vi "NodeID to Section Pointer.vi"(8 "error in (no error)":errorcluster, 11 "nodeID in":T1 format="%.0x") -> (0 "error out":errorcluster, 2 "BaseNodeType out":refnum<k24>, 3 "nodeID out":T1 format="%.0x")   [LabVIEW 2023, in "Instrument Addon Scripting API.lvlib"]
uses:
  Instrument Addon Scripting API.lvlib
  <vilib>/NI VeriStand/Custom Device API/Custom Device Item Ref.ctl
  NationalInstruments.VeriStand.SystemStorage
  NationalInstruments.VeriStand.SystemDefinitionAPI
  <vilib>/NI VeriStand/Custom Device API/Custom Device API.lvlib
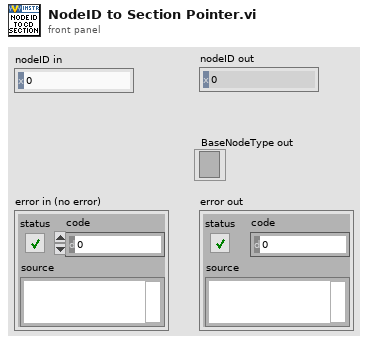
[diagram p1: front panel]
types:
  T1 = typedef "Custom Device API.lvlib/Custom Device Item Ref.ctl" = u64
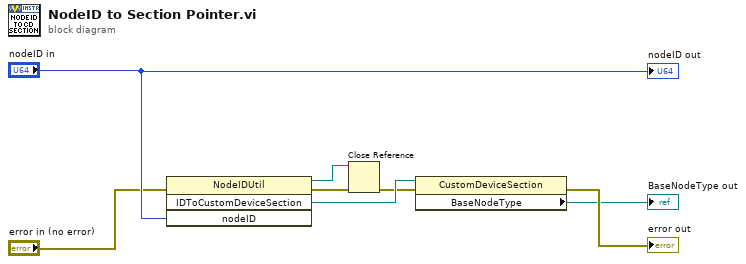
[diagram p0: block diagram]
diagram:
  n1 = invoke class="NodeIDUtil" method="IDToCustomDeviceSection"(error in="error in (no error)", "nodeID"="nodeID in") -> (reference out=w2:refnum<k24>, error out=w3:errorcluster, "IDToCustomDeviceSection"=w4:refnum<k24>)  [unwired: 2 in, 1 out]
  n2 = Close Reference(reference=w2, error in (no error)=w3) -> (error out=w1:errorcluster)
  n3 = property class="CustomDeviceSection"(reference=w4, error in=w1) -> (error out=→"error out":errorcluster, "BaseNodeType"=→"BaseNodeType out":refnum<k24>)  [unwired: 1 out]
  "nodeID out" <- "nodeID in"
